vi "LoadRebootCounts.vi"(8 "error in (no error)":errorcluster, 10 "lookback minutes":i32, 11 "log dir":path) -> (0 "error out":errorcluster, 2 "reboot count":i32, 3 "log dir":path)   [LabVIEW 2017, in "Controller.lvlib"]
uses:
  <vilib>/addons/InsightCM/Devices/Shared/Common/Controller/Controller.lvlib
  <vilib>/addons/InsightCM/Devices/Shared/Common/Controller/controls/operations.ctl
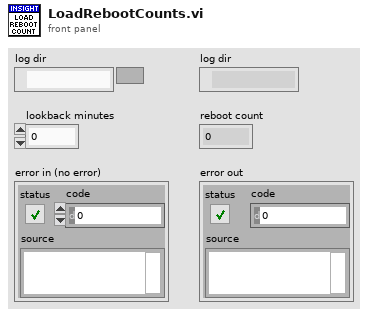
[diagram p1: front panel]
types:
  T1 = typedef "Controller.lvlib/operations.ctl" = enum16{"Unknown", "Startup", "Expected Shutdown"}
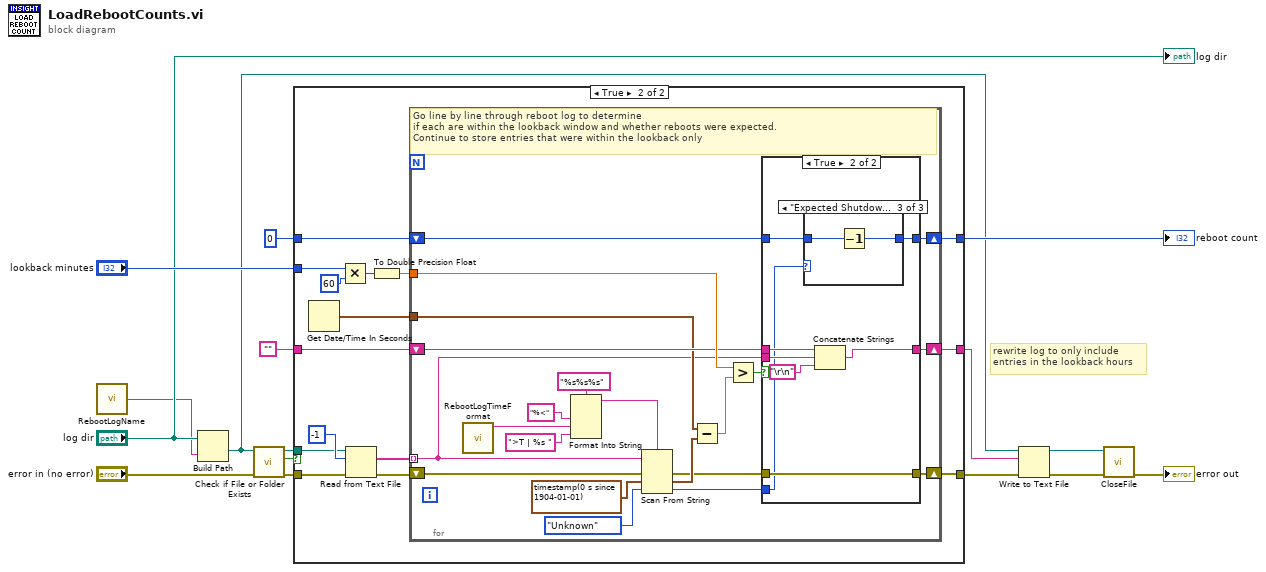
[diagram p0: block diagram]
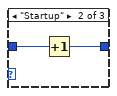
[diagram p5: hidden frame]
diagram:
  # "rewrite log to only include \nentries in the lookback hours"
  n1 = call <vilib>:"RebootLogName.vi"() -> ("reboot log name"=w12:string)  [unwired: 5 in]
  n2 = Build Path(base path="log dir", name or relative path=w12) -> (appended path=w4:path)
  n3 = call <vilib>:"Check if File or Folder Exists.vi"("error in (no error)"="error in (no error)", "path"=w4) -> ("error out"=w9:errorcluster, "file or folder exists?"=w10:bool, "dup path"=w11:path)  [unwired: 7 in]
  n4 = case shown="True" w10 {
    tunnel: [w19 w34] -> w6
    tunnel: w9 -> [w19 w28]
    tunnel: w11 -> [_ w25]
    tunnel: "lookback minutes" -> [_ w22]
    tunnel: [w18 w33] -> w16
    tunnel: 0 -> [w18 w32]
    tunnel: "" -> [w17 w31]
    tunnel: [w17 w30] -> w5
    frame False {
    }
    frame True {
      n5 = Get Date/Time In Seconds() -> (seconds since 1Jan1904=w29:timestamp)
      n6 = Multiply(x=w22, y=60) -> (x*y=w23:i32)
      n7 = Read from Text File(file (use dialog)=w25, count=-1, error in=w28) -> (text=w24:string[], error out=w27:errorcluster)  [unwired: 1 in, 2 out]
      n8 = To Double Precision Float(number=w23) -> (double precision float=w20:dbl)
      n9 = for {
        shift-right: [w52] -> w34
        shift-left: w27 -> [w48]
        tunnel: w20 -> [w55]
        shift-right: [w53] -> w33
        shift-left: w32 -> [w54]
        shift-right: [w50] -> w30
        shift-left: w31 -> [w51]
        tunnel: w29 -> [w49]
        tunnel: w24 -> [w43] mode=indexing
        # "Go line by line through reboot log to determine\nif each are within the lookback window and whether reboots were expected. \nContinue to store entries that were within the lookback only"
        n10 = call <vilib>:"RebootLogTimeFormat.vi"() -> ("time format"=w35:string)  [unwired: 11 in]
        n11 = Format Into String(format string="%s%s%s", "%<" ("format string"), w35, ">T | %s " ("format string")) -> (resulting string=w36:string)  [unwired: 2 in, 1 out]
        n12 = Scan From String(format string=w36, input string=w43, error in=w48, default 1=timestamp(0 s since 1904-01-01) ("current time"), default 2=operations."Unknown") -> (error out=w44:errorcluster, output 1=w47:timestamp, output 2=w41:T1)  [unwired: 1 in, 2 out]
        n13 = Subtract(x=w49, y=w47) -> (x-y=w46:dbl)
        n14 = Greater?(x=w55, y=w46) -> (0:w45:bool)
        n15 = case shown="True" w45 {
          tunnel: w44 -> [w58 w66]
          tunnel: [w58 w66] -> w52
          tunnel: w54 -> [w57 w63]
          tunnel: [w57 w62] -> w53
          tunnel: [w56 w64] -> w50
          tunnel: w51 -> [w56 w65]
          tunnel: w43 -> [_ w61]
          tunnel: w41 -> [_ w59]
          frame False {
          }
          frame True {
            n16 = case shown="\"Expected Shutdown\"" w59 {
              tunnel: w63 -> [w67 w69 w71]
              tunnel: [w67 w68 w70] -> w62
              frame Default {
              }
              frame "Startup" {
                n17 = Increment(x=w69) -> (x+1=w68:i32)
              }
              frame "Expected Shutdown" {
                n18 = Decrement(x=w71) -> (x-1=w70:i32)
              }
            }
            n19 = Concatenate Strings(w65, w61, "\r\n") -> (w64:string)
          }
        }
      }
    }
  }
  "reboot count" <- w16
  n20 = Write to Text File(file (use dialog)=w4, text=w5, error in=w6) -> (refnum out=w3:refnum<file>, error out=w2:errorcluster)  [unwired: 1 in, 1 out]
  n21 = call <vilib>:"CloseFile.vi"("error in (no error)"=w2, "file reference"=w3) -> ("error out"=→"error out":errorcluster)  [unwired: 9 in]
  "log dir" <- "log dir"
